vi "XML_EEG_readDataset.vi"(8 "error in (no error)":errorcluster, 9 "Add offset?":bool, 10 "DatasetNumber":i32, 11 "XML_EEG_File in":refnum<class "XML_EEG_File.lvclass">) -> (1 "Errors?":bool, 2 "XML Dataset out":T1, 3 "XML_EEG_File out":refnum<class "XML_EEG_File.lvclass">)   [LabVIEW 2016, in "XML_EEG_File_Parser.lvlib" / "XML_EEG_File.lvclass"]
uses:
  XML_EEG_File.lvclass
  XML_EEG_Dataset.ctl
  XML_EEG_File.lvclass/XML_EEG_File.ctl
  <vilib>/Waveform/WDTOps.llb/WDT Number of Waveform Samples DBL.vi
  <vilib>/xml/NI_XML.lvlib
  XML_EEG_File_Parser.lvlib
panel:
  # "This VI is a part of BCI Design library, http://www.ru-bci.org \nCopyright © 2020, Sotnikov Peter, All rights reserved. License: GNU GPLv3"
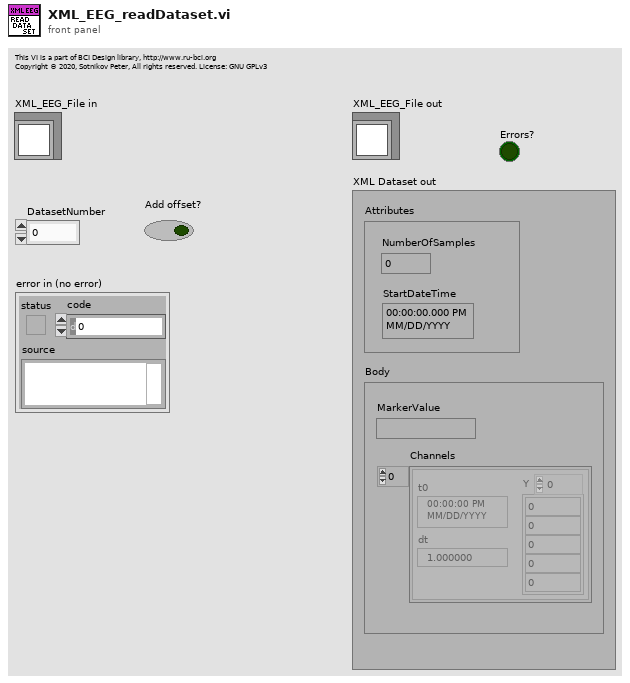
[diagram p1: front panel]
types:
  T1 = typedef "XML_EEG_File_Parser.lvlib/XML_EEG_Dataset.ctl" = cluster{"Attributes":cluster{"NumberOfSamples":i32, "StartDateTime":timestamp}, "Body":cluster{"MarkerValue":string, "Channels":waveform(dbl)[]}}
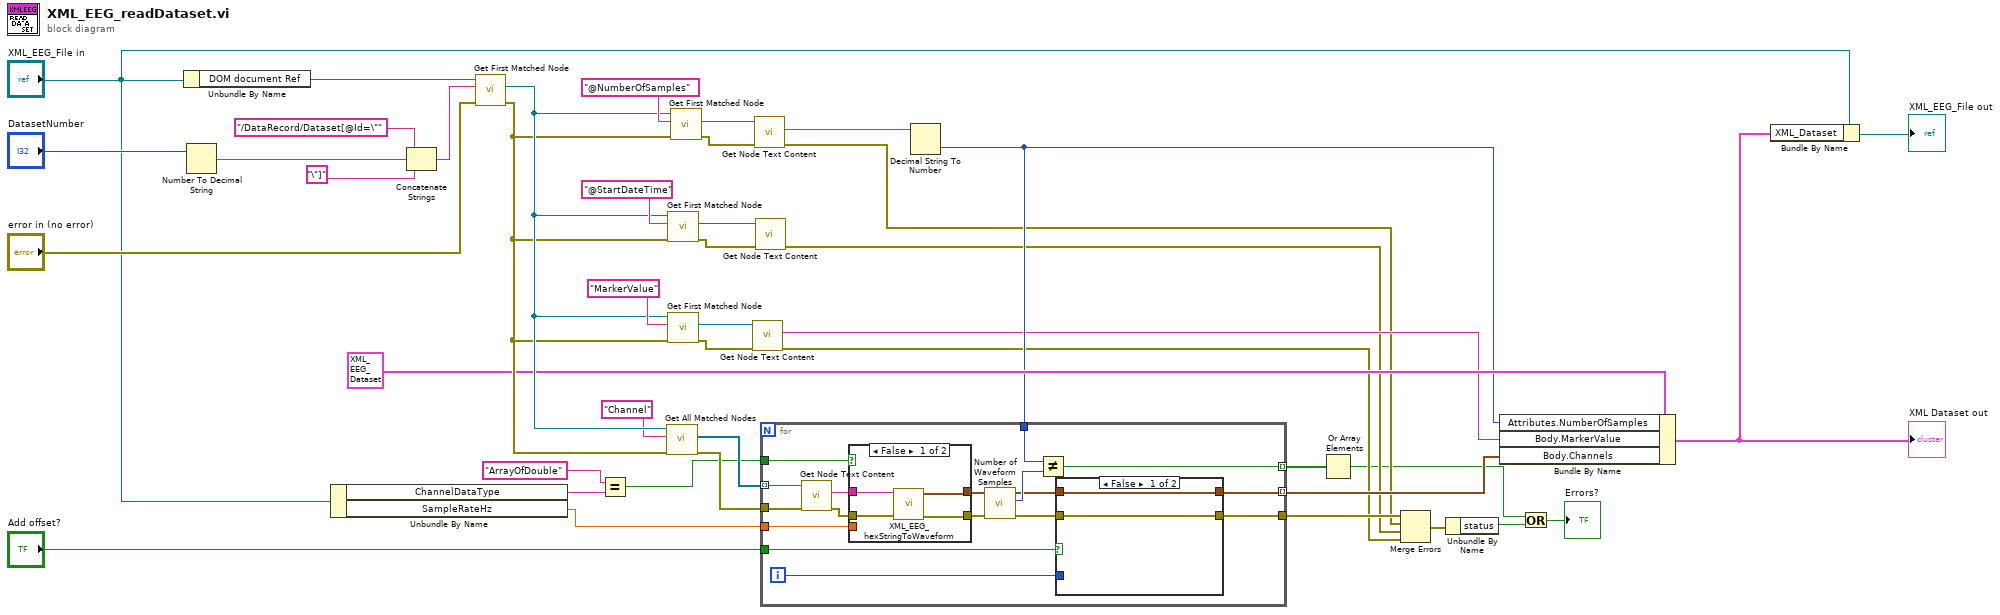
[diagram p0: block diagram]
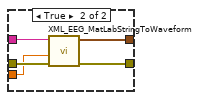
[diagram p2: hidden frame]
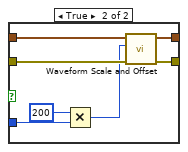
[diagram p3: hidden frame]
diagram:
  n1 = Unbundle By Name("XML_EEG_File in") -> ("DOM document Ref"=w8:refnum<k20>)
  n2 = Number To Decimal String(number="DatasetNumber") -> (decimal integer string=w40:string)  [unwired: 1 in]
  n3 = Unbundle By Name("XML_EEG_File in") -> ("ChannelDataType"=w4:string, "SampleRateHz"=w1:dbl)
  n4 = Concatenate Strings("/DataRecord/Dataset[@Id=\"" ("XPath expression"), w40, "\"]" ("XPath expression")) -> (w39:string)
  n5 = call <vilib>:"Get First Matched Node.vi"("error in (no error)"="error in (no error)", "XPath expression"=w39, "node in"=w8) -> ("error out"=w27:errorcluster, "node result"=w28:refnum<k20>)  [unwired: 6 in, 1 out]
  n6 = Equal?(x="ArrayOfDouble", y=w4) -> (x = y?=w2:bool)
  n7 = call <vilib>:"Get All Matched Nodes.vi"("error in (no error)"=w27, "XPath expression"="Channel", "node in"=w28) -> ("error out"=w23:errorcluster, "node result array"=w24:refnum<k20>[])  [unwired: 6 in, 1 out]
  n8 = call <vilib>:"Get First Matched Node.vi"("error in (no error)"=w27, "XPath expression"="@StartDateTime", "node in"=w28) -> ("error out"=w32:errorcluster, "node result"=w33:refnum<k20>)  [unwired: 6 in, 1 out]
  n9 = call <vilib>:"Get First Matched Node.vi"("error in (no error)"=w27, "XPath expression"="MarkerValue", "node in"=w28) -> ("error out"=w29:errorcluster, "node result"=w30:refnum<k20>)  [unwired: 6 in, 1 out]
  n10 = call <vilib>:"Get First Matched Node.vi"("error in (no error)"=w27, "XPath expression"="@NumberOfSamples", "node in"=w28) -> ("error out"=w35:errorcluster, "node result"=w36:refnum<k20>)  [unwired: 6 in, 1 out]
  n11 = call <vilib>:"Get Node Text Content.vi"("error in (no error)"=w29, "node in"=w30) -> ("error out"=w14:errorcluster, "node text"=w19:string)  [unwired: 7 in, 1 out]
  n12 = call <vilib>:"Get Node Text Content.vi"("error in (no error)"=w35, "node in"=w36) -> ("error out"=w16:errorcluster, "node text"=w25:string)  [unwired: 7 in, 1 out]
  n13 = call <vilib>:"Get Node Text Content.vi"("error in (no error)"=w32, "node in"=w33) -> ("error out"=w15:errorcluster)  [unwired: 7 in, 2 out]
  n14 = Decimal String To Number(string=w25) -> (number=w20:i32)  [unwired: 2 in, 1 out]
  n15 = for {
    tunnel: w24 -> [w60] mode=indexing
    tunnel: w23 -> [w59]
    tunnel: w20 -> [w53]
    tunnel: [w50] -> w18 mode=indexing
    tunnel: [w52] -> w22 mode=indexing
    tunnel: [w48] -> w17
    tunnel: "Add offset?" -> [w47]
    tunnel: w2 -> [w45]
    tunnel: w1 -> [w44]
    i -> [w46]
    n16 = call <vilib>:"Get Node Text Content.vi"("error in (no error)"=w59, "node in"=w60) -> ("error out"=w57:errorcluster, "node text"=w58:string)  [unwired: 7 in, 1 out]
    n17 = case shown="False" w45 {
      tunnel: w58 -> [w63 w69]
      tunnel: w57 -> [w64 w68]
      tunnel: [w61 w67] -> w56
      tunnel: [w62 w66] -> w55
      tunnel: w44 -> [_ w65]
      frame False {
        n18 = call "XML_EEG_hexStringToWaveform.vi"("error in (no error)"=w64, "Hex String in"=w63) -> ("error out"=w61:errorcluster, "Waveform out"=w62:waveform(dbl))  [unwired: 8 in]
      }
      frame True {
        n19 = call "XML_EEG_MatLabStringToWaveform.vi"("error in (no error)"=w68, "SampleRateHz"=w65, "Hex String in"=w69) -> ("error out"=w67:errorcluster, "Waveform out"=w66:waveform(dbl))  [unwired: 7 in]
      }
    }
    n20 = call-poly <vilib>:"Number of Waveform Samples.vi"("error in (no error)"=w56, "waveform in"=w55) -> ("error out"=w49:errorcluster, "number of samples"=w54:i32, "waveform out"=w51:waveform(dbl))  [unwired: 7 in]
    n21 = Not Equal?(x=w53, y=w54) -> (x != y?=w52:bool)
    n22 = case shown="False" w47 {
      tunnel: w51 -> [w71 w76]
      tunnel: [w71 w77] -> w50
      tunnel: w49 -> [w70 w75]
      tunnel: [w70 w78] -> w48
      tunnel: w46 -> [_ w74]
      frame False {
      }
      frame True {
        n23 = Multiply(x=200, y=w74) -> (x*y=w72:i32)
        n24 = call <vilib>:"Waveform Scale and Offset.vi"("error in (no error)"=w75, "offset"=w72, "waveform in"=w76) -> ("error out"=w78:errorcluster, "waveform out"=w77:waveform(dbl))  [unwired: 7 in]
      }
    }
  }
  n25 = Or Array Elements(Boolean array=w22) -> (logical OR=w10:bool)
  n26 = Merge Errors(w17, w16, w15, w14) -> (w13:errorcluster)
  n27 = Unbundle By Name(w13) -> ("status"=w12:bool)
  n28 = Bundle By Name(cluster=T1 {"Attributes"={"NumberOfSamples"=0, "StartDateTime"=timestamp(0 s since 1904-01-01)}, "Body"={"MarkerValue"="", "Channels"=[]}} ("XML_Dataset"), "Attributes.NumberOfSamples"=w20, "Body.MarkerValue"=w19, "Body.Channels"=w18) -> (w7:T1)
  "XML Dataset out" <- w7
  n29 = Or(x=w10, y=w12) -> (x .or. y?=→"Errors?":bool)
  n30 = Bundle By Name(cluster="XML_EEG_File in", "XML_Dataset"=w7) -> (→"XML_EEG_File out":refnum<class "XML_EEG_File.lvclass">)
